vi "lock.vi"() -> ()   [LabVIEW 2022 SP3]
panel:
  out "error out 8":errorcluster
  out "error out 7":errorcluster
  out "error out 2":errorcluster
  out "error out":errorcluster
  out "error out 3":errorcluster
  out "error out 4":errorcluster
  out "error out 5":errorcluster
  out "error out 6":errorcluster
  in  "Tab Control":enum32{"Page 1", "Page 2"}(tab)
  in  "Refresh Button":bool
  in  "ENTER PIN":string
  in  "stop":bool
  out "text":string
  in  "?":bool
  out "1":dbl
  out "2":dbl
  out "3":dbl
  out "4":dbl
  out "5":dbl
  out "6":dbl
  out "7":dbl
  out "8":dbl
  out "8 2":dbl
  out "7 2":dbl
  # "MAX"
  # "MIN"
  # "400"
  # "320"
  # "240"
  # "210"
  # "180"
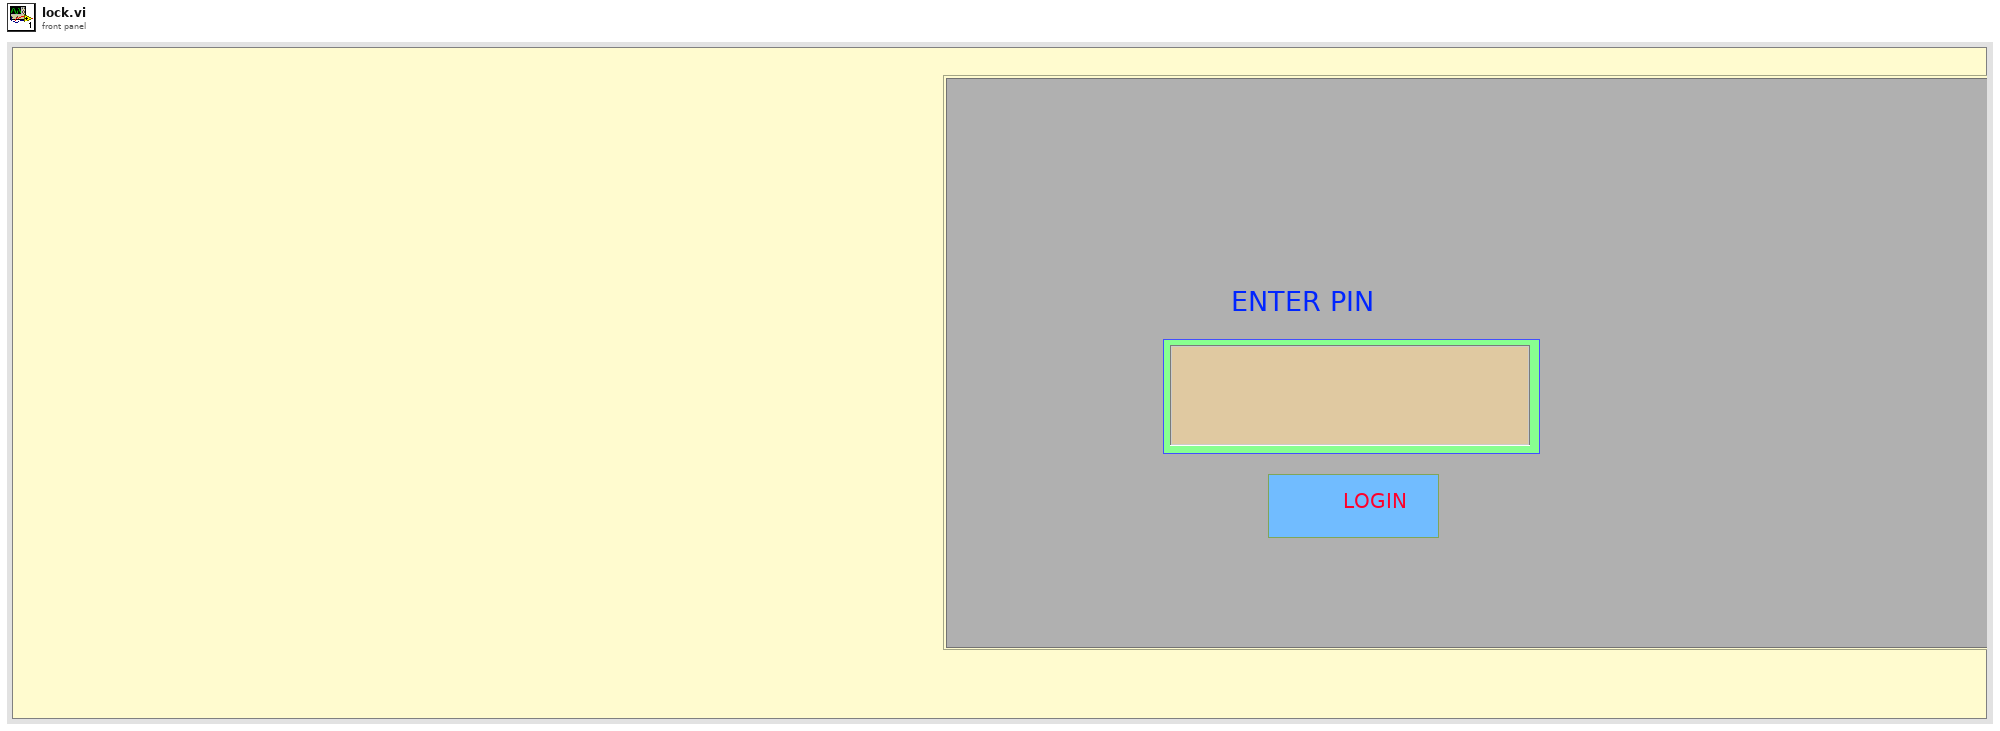
[diagram p1: front panel]
types:
  T1 = enum16{"open", "replace", "create", "open or create", "replace or create", "replace or create with confirmation"}
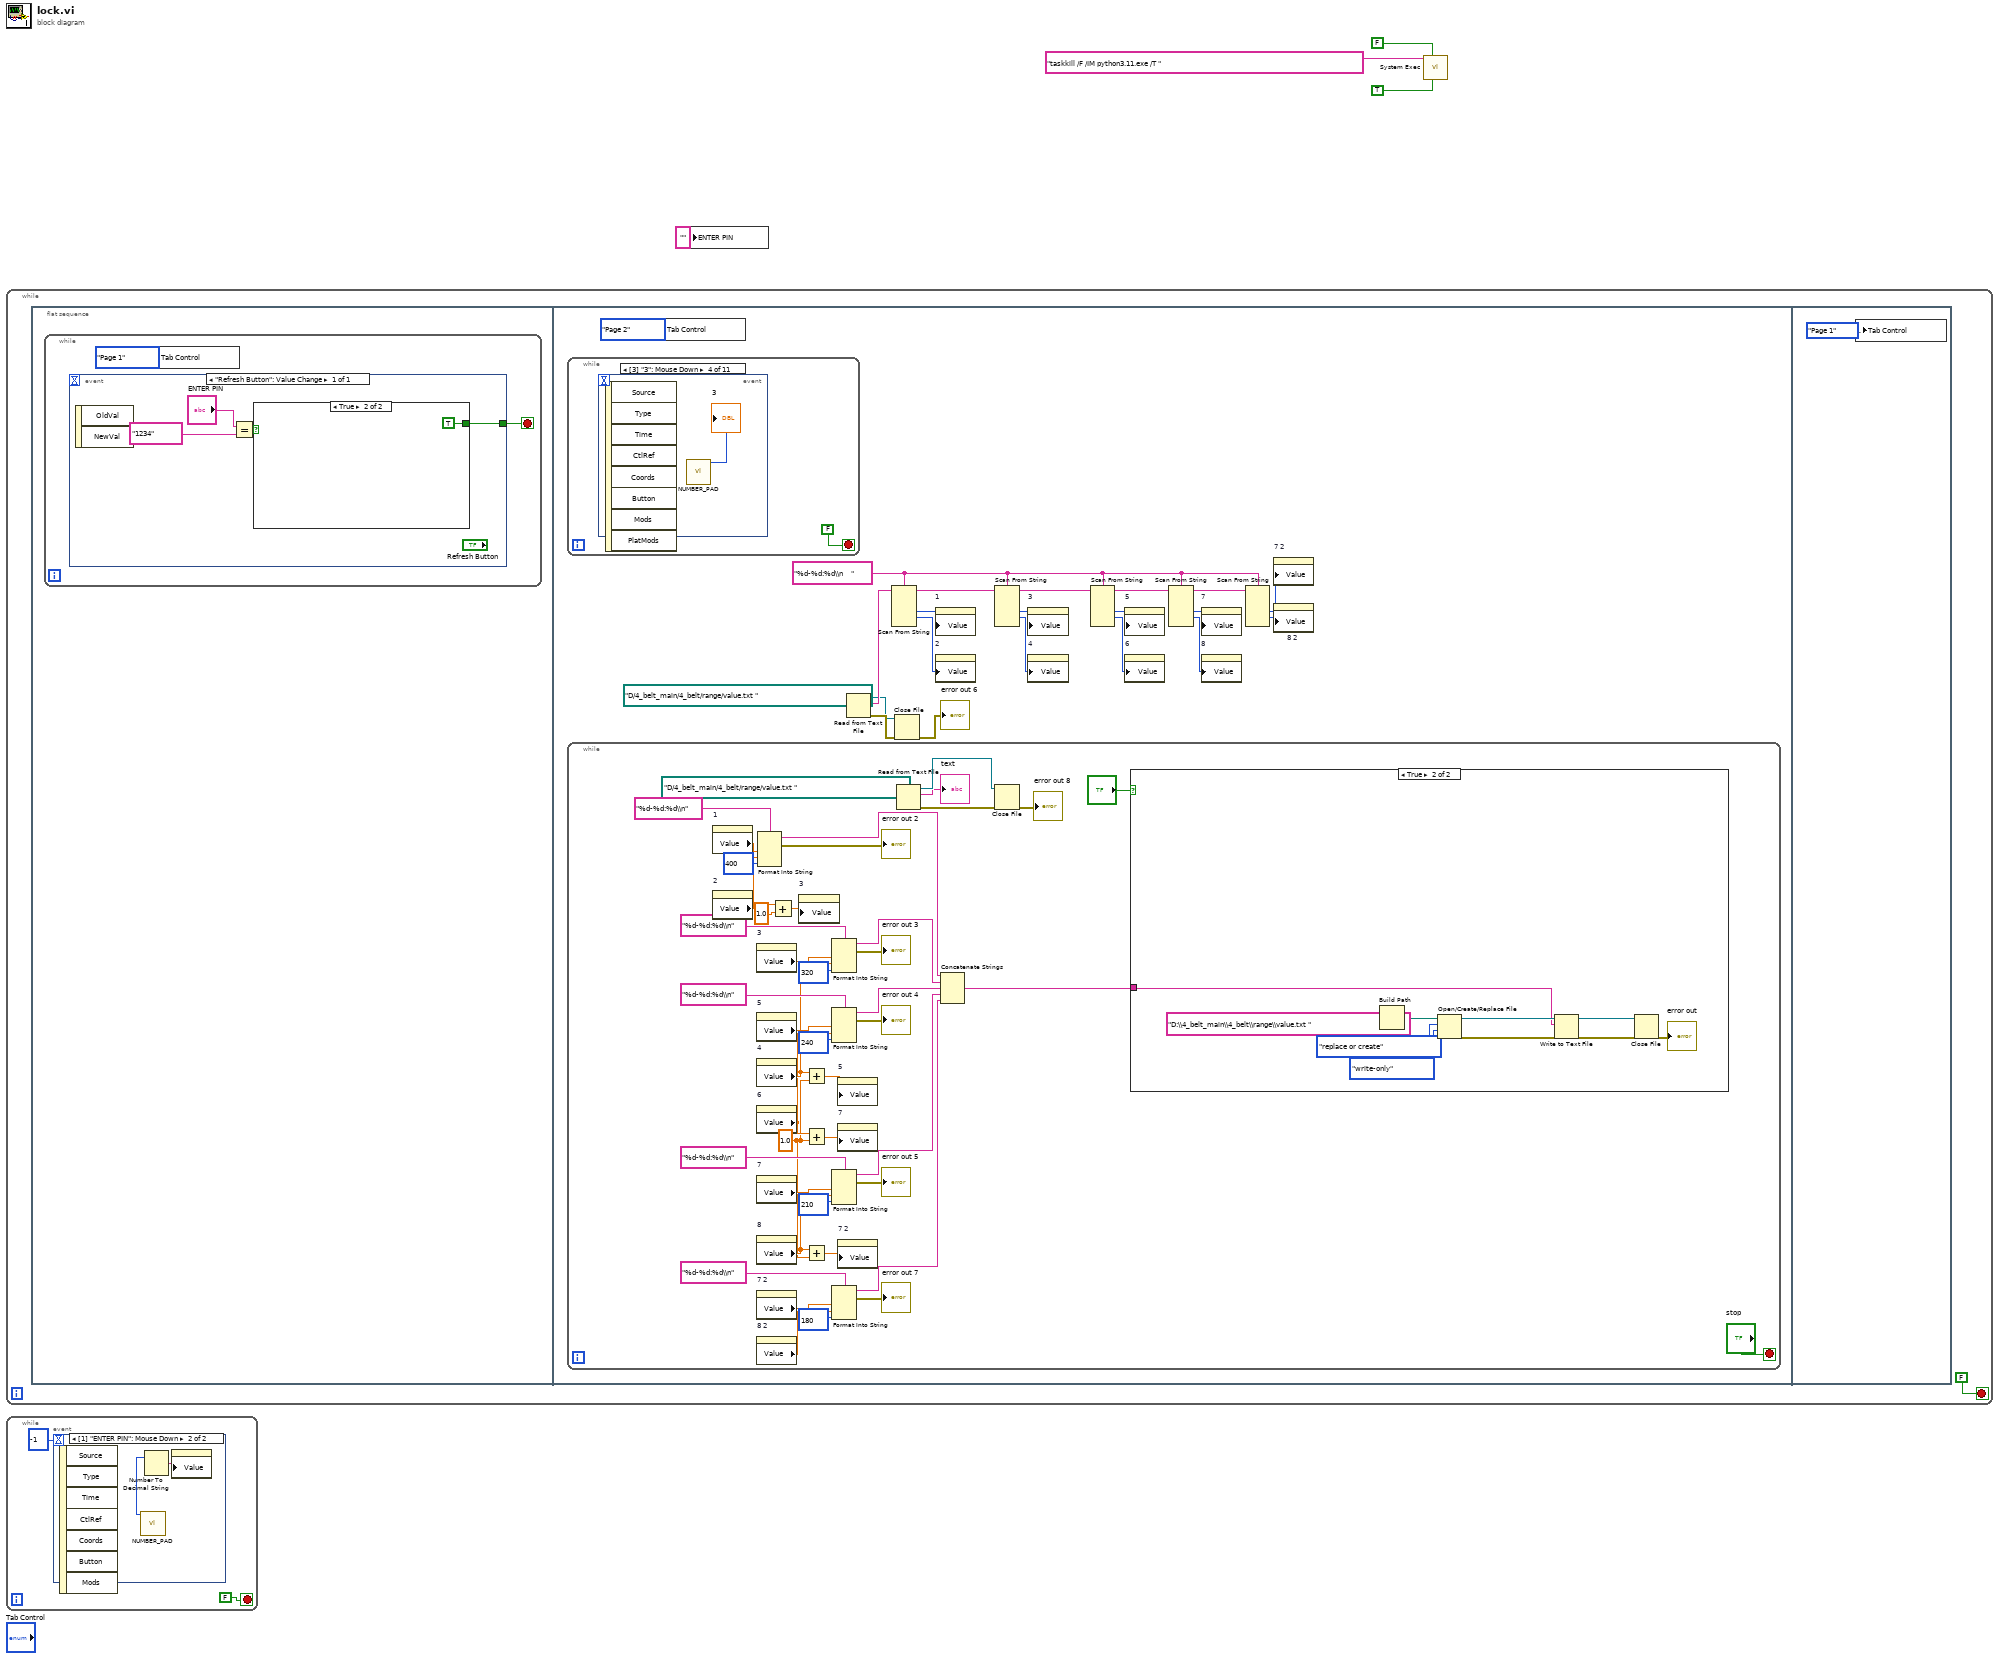
[diagram p0: block diagram]
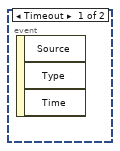
[diagram p2: hidden frame]
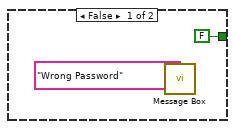
[diagram p3: hidden frame]
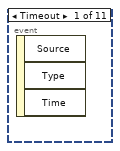
[diagram p4: hidden frame]
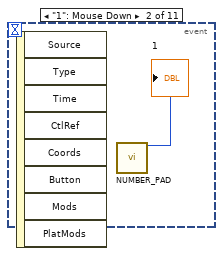
[diagram p5: hidden frame]
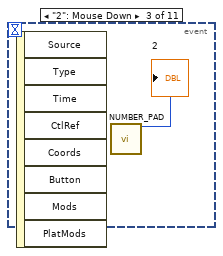
[diagram p6: hidden frame]
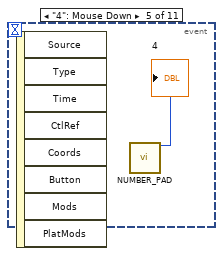
[diagram p7: hidden frame]
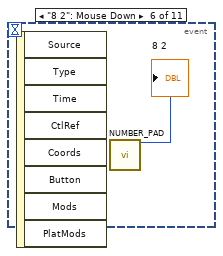
[diagram p8: hidden frame]
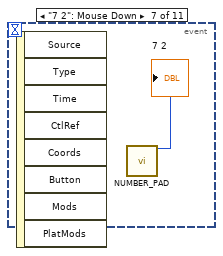
[diagram p9: hidden frame]
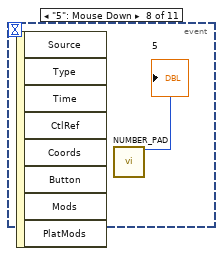
[diagram p10: hidden frame]
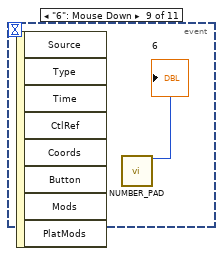
[diagram p11: hidden frame]
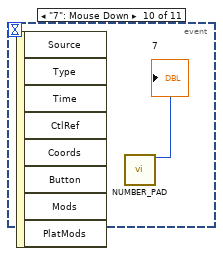
[diagram p12: hidden frame]
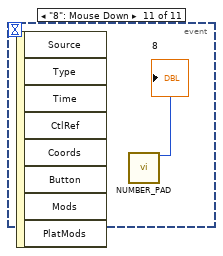
[diagram p13: hidden frame]
diagram:
  n1 = while {
    stop <- FALSE stop-if-true
    n2 = flat-sequence {
      frame #0 {
        n3 = while {
          stop <- w7 stop-if-true
          n4 = event shown="[0] \"Refresh Button\": Value Change" {
            selector: _ -> [_]
            dyn-events: _ -> [_]
            timeout: _ -> [_]
            tunnel: [w9] -> w7
            event "Refresh Button": Value Change {
              n5 = event-data() -> ()  [unwired: 1 in, 2 out]
              n6 = Equal?(x="ENTER PIN", y="1234") -> (x = y?=w8:bool)
              n7 = case shown="True" w8 {
                tunnel: [FALSE TRUE] -> w9
                frame False {
                  n8 = call "Message Box.vi"("String"="Wrong Password") -> ()  [unwired: 9 in, 1 out]
                }
                frame True {
                }
              }
            }
          }
          n9 = local write "Tab Control"(enum32{"Page 1", "Page 2"}."Page 1" ("Tab Control")) -> ()
        }
      }
      frame #1 {
        w17 = "%d-%d:%d\\n    " ("format string")
        n10 = while {
          stop <- FALSE stop-if-true
          n11 = event shown="[3] \"3\": Mouse Down" {
            selector: _ -> [_ _ _ _ _ _ _ _ _ _ _]
            dyn-events: _ -> [_ _ _ _ _ _ _ _ _ _ _]
            timeout: _ -> [_ _ _ _ _ _ _ _ _ _ _]
            event Timeout {
              n12 = event-data() -> ()  [unwired: 1 in, 3 out]
            }
            event "1": Mouse Down {
              n13 = event-data() -> ()  [unwired: 1 in, 8 out]
              n14 = call "NUMBER_PAD.vi"() -> ("number (out)"=→"1":i32)  [unwired: 15 in]
            }
            event "2": Mouse Down {
              n15 = event-data() -> ()  [unwired: 1 in, 8 out]
              n16 = call "NUMBER_PAD.vi"() -> ("number (out)"=→"2":i32)  [unwired: 15 in]
            }
            event "3": Mouse Down {
              n17 = event-data() -> ()  [unwired: 1 in, 8 out]
              n18 = call "NUMBER_PAD.vi"() -> ("number (out)"=→"3":i32)  [unwired: 15 in]
            }
            event "4": Mouse Down {
              n19 = event-data() -> ()  [unwired: 1 in, 8 out]
              n20 = call "NUMBER_PAD.vi"() -> ("number (out)"=→"4":i32)  [unwired: 15 in]
            }
            event "8 2": Mouse Down {
              n21 = event-data() -> ()  [unwired: 1 in, 8 out]
              n22 = call "NUMBER_PAD.vi"() -> ("number (out)"=→"8 2":i32)  [unwired: 15 in]
            }
            event "7 2": Mouse Down {
              n23 = event-data() -> ()  [unwired: 1 in, 8 out]
              n24 = call "NUMBER_PAD.vi"() -> ("number (out)"=→"7 2":i32)  [unwired: 15 in]
            }
            event "5": Mouse Down {
              n25 = event-data() -> ()  [unwired: 1 in, 8 out]
              n26 = call "NUMBER_PAD.vi"() -> ("number (out)"=→"5":i32)  [unwired: 15 in]
            }
            event "6": Mouse Down {
              n27 = event-data() -> ()  [unwired: 1 in, 8 out]
              n28 = call "NUMBER_PAD.vi"() -> ("number (out)"=→"6":i32)  [unwired: 15 in]
            }
            event "7": Mouse Down {
              n29 = event-data() -> ()  [unwired: 1 in, 8 out]
              n30 = call "NUMBER_PAD.vi"() -> ("number (out)"=→"7":i32)  [unwired: 15 in]
            }
            event "8": Mouse Down {
              n31 = event-data() -> ()  [unwired: 1 in, 8 out]
              n32 = call "NUMBER_PAD.vi"() -> ("number (out)"=→"8":i32)  [unwired: 15 in]
            }
          }
        }
        n33 = while {
          stop <- "stop" stop-if-true
          w54 = 1.0 ("y")
          n34 = property on="1" class="DigNum (strict)"() -> ("Value"=w72:dbl)  [unwired: 2 in, 2 out]
          n35 = property on="2" class="DigNum (strict)"() -> ("Value"=w62:dbl)  [unwired: 2 in, 2 out]
          n36 = property on="3" class="DigNum (strict)"() -> ("Value"=w71:dbl)  [unwired: 2 in, 2 out]
          n37 = property on="5" class="DigNum (strict)"() -> ("Value"=w70:dbl)  [unwired: 2 in, 2 out]
          n38 = property on="4" class="DigNum (strict)"() -> ("Value"=w58:dbl)  [unwired: 2 in, 2 out]
          n39 = property on="6" class="DigNum (strict)"() -> ("Value"=w57:dbl)  [unwired: 2 in, 2 out]
          n40 = property on="7" class="DigNum (strict)"() -> ("Value"=w69:dbl)  [unwired: 2 in, 2 out]
          n41 = property on="8" class="DigNum (strict)"() -> ("Value"=w55:dbl)  [unwired: 2 in, 2 out]
          n42 = property on="7 2" class="DigNum (strict)"() -> ("Value"=w64:dbl)  [unwired: 2 in, 2 out]
          n43 = property on="8 2" class="DigNum (strict)"() -> ("Value"=w63:dbl)  [unwired: 2 in, 2 out]
          n44 = Format Into String "Format Into String"(format string="%d-%d:%d\\n", w72, w62, 400) -> (resulting string=w86:string, error out=→"error out 2":errorcluster)  [unwired: 2 in]
          n45 = Add(x=w62, y=1.0) -> (x+y=w60:dbl)
          n46 = property on="3" class="DigNum (strict)"("Value"=w60) -> ()  [unwired: 2 in, 2 out]
          n47 = Add(x=w58, y=w54) -> (x+y=w59:dbl)
          n48 = Add(x=w57, y=w54) -> (x+y=w56:dbl)
          n49 = Add(x=w55, y=w54) -> (x+y=w53:dbl)
          n50 = Format Into String(format string="%d-%d:%d\\n", w71, w58, 320) -> (resulting string=w84:string, error out=→"error out 3":errorcluster)  [unwired: 2 in]
          n51 = Format Into String(format string="%d-%d:%d\\n", w70, w57, 240) -> (resulting string=w78:string, error out=→"error out 4":errorcluster)  [unwired: 2 in]
          n52 = Format Into String(format string="%d-%d:%d\\n", w69, w55, 210) -> (resulting string=w77:string, error out=→"error out 5":errorcluster)  [unwired: 2 in]
          n53 = Format Into String(format string="%d-%d:%d\\n", w64, w63, 180) -> (resulting string=w65:string, error out=→"error out 7":errorcluster)  [unwired: 2 in]
          n54 = property on="5" class="DigNum (strict)"("Value"=w59) -> ()  [unwired: 2 in, 2 out]
          n55 = property on="7" class="DigNum (strict)"("Value"=w56) -> ()  [unwired: 2 in, 2 out]
          n56 = property on="7 2" class="DigNum (strict)"("Value"=w53) -> ()  [unwired: 2 in, 2 out]
          n57 = Read from Text File(file (use dialog)=path "D:/4_belt_main/4_belt/range/value.txt ") -> (refnum out=w51:refnum<file>, text=→"text":string, error out=w50:errorcluster)  [unwired: 3 in, 1 out]
          n58 = Concatenate Strings "Concatenate Strings"(w86, w84, w78, w77, w65) -> (w73:string)
          n59 = Close File(refnum=w51, error in=w50) -> (error out=→"error out 8":errorcluster)  [unwired: 1 out]
          n60 = case shown="True" "?" {
            tunnel: w73 -> [_ w94]
            frame False {
            }
            frame True {
              n61 = Build Path(name or relative path="D:\\4_belt_main\\4_belt\\range\\value.txt ") -> (appended path=w98:path)  [unwired: 1 in]
              n62 = Open/Create/Replace File(file path (use dialog)=w98, operation (0:open)=T1."replace or create", access (0:read/write)=enum16{"read/write", "read-only", "write-only"}."write-only") -> (refnum out=w95:refnum<file>, error out=w96:errorcluster)  [unwired: 3 in, 1 out]
              n63 = Write to Text File(file (use dialog)=w95, text=w94, error in=w96) -> (refnum out=w93:refnum<file>, error out=w92:errorcluster)  [unwired: 1 in, 1 out]
              n64 = Close File(refnum=w93, error in=w92) -> (error out=→"error out":errorcluster)  [unwired: 1 out]
            }
          }
        }
        n65 = local write "Tab Control"(enum32{"Page 1", "Page 2"}."Page 2" ("Tab Control")) -> ()
        n66 = Read from Text File(file (use dialog)=path "D:/4_belt_main/4_belt/range/value.txt ") -> (refnum out=w18:refnum<file>, text=w21:string, error out=w19:errorcluster)  [unwired: 3 in, 1 out]
        n67 = Scan From String(format string=w17, input string=w21) -> (remaining string=w22:string, output 1=w23:i32, output 2=w24:i32)  [unwired: 6 in, 2 out]
        n68 = Close File(refnum=w18, error in=w19) -> (error out=→"error out 6":errorcluster)  [unwired: 1 out]
        n69 = property on="1" class="DigNum (strict)"("Value"=w23) -> ()  [unwired: 2 in, 2 out]
        n70 = property on="2" class="DigNum (strict)"("Value"=w24) -> ()  [unwired: 2 in, 2 out]
        n71 = Scan From String(format string=w17, input string=w22) -> (remaining string=w32:string, output 1=w25:i32, output 2=w26:i32)  [unwired: 6 in, 2 out]
        n72 = property on="3" class="DigNum (strict)"("Value"=w25) -> ()  [unwired: 2 in, 2 out]
        n73 = property on="4" class="DigNum (strict)"("Value"=w26) -> ()  [unwired: 2 in, 2 out]
        n74 = Scan From String(format string=w17, input string=w32) -> (remaining string=w33:string, output 1=w27:i32, output 2=w28:i32)  [unwired: 6 in, 2 out]
        n75 = property on="5" class="DigNum (strict)"("Value"=w27) -> ()  [unwired: 2 in, 2 out]
        n76 = property on="6" class="DigNum (strict)"("Value"=w28) -> ()  [unwired: 2 in, 2 out]
        n77 = Scan From String(format string=w17, input string=w33) -> (remaining string=w34:string, output 1=w29:i32, output 2=w30:i32)  [unwired: 6 in, 2 out]
        n78 = property on="7" class="DigNum (strict)"("Value"=w29) -> ()  [unwired: 2 in, 2 out]
        n79 = property on="8" class="DigNum (strict)"("Value"=w30) -> ()  [unwired: 2 in, 2 out]
        n80 = Scan From String(format string=w17, input string=w34) -> (output 1=w31:i32, output 2=w15:i32)  [unwired: 6 in, 3 out]
        n81 = property on="7 2" class="DigNum (strict)"("Value"=w31) -> ()  [unwired: 2 in, 2 out]
        n82 = property on="8 2" class="DigNum (strict)"("Value"=w15) -> ()  [unwired: 2 in, 2 out]
      }
      frame #2 {
        n83 = local write "Tab Control"(enum32{"Page 1", "Page 2"}."Page 1" ("Tab Control")) -> ()
      }
    }
  }
  n84 = while {
    stop <- FALSE stop-if-true
    n85 = event shown="[1] \"ENTER PIN\": Mouse Down" {
      selector: _ -> [_ _]
      dyn-events: _ -> [_ _]
      timeout: -1 -> [_ _]
      event Timeout {
        n86 = event-data() -> ()  [unwired: 1 in, 3 out]
      }
      event "ENTER PIN": Mouse Down {
        n87 = event-data() -> ()  [unwired: 1 in, 7 out]
        n88 = call "NUMBER_PAD.vi"() -> ("number (out)"=w104:i32)  [unwired: 15 in]
        n89 = Number To Decimal String(number=w104) -> (decimal integer string=w105:string)  [unwired: 1 in]
        n90 = property on="ENTER PIN" class="Str"("Value"=w105) -> ()  [unwired: 2 in, 2 out]
      }
    }
  }
  n91 = local write "ENTER PIN"("" ("ENTER PIN")) -> ()
  n92 = call <vilib>:"System Exec.vi"("run minimized? (F)"=TRUE, "wait until completion? (T)"=FALSE, "command line"="taskkill /F /IM python3.11.exe /T ") -> ()  [unwired: 5 in, 4 out]
